vi "Remove Messages and Subaddresses.vi"(8 "error in":errorcluster, 11 "messages or subaddresses":T1[](array[typedef]) format="%.0x") -> (0 "error out":errorcluster)   [LabVIEW 2020, in "AIM MIL-STD-1553 Scripting.lvlib"]
doc: "Removes the specified <b>messages or subaddresses</b> from their parent system definition. Once the references have been removed, they are no longer valid. This VI will return an error if called to remove invalid references."
uses:
  AIM MIL-STD-1553 Scripting.lvlib
  <vilib>/NI VeriStand/Custom Device API/Custom Device Item Ref.ctl
  <vilib>/NI VeriStand/Custom Device API/Custom Device API.lvlib
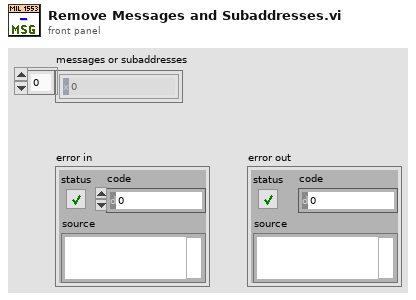
[diagram p1: front panel]
types:
  T1 = typedef "Custom Device API.lvlib/Custom Device Item Ref.ctl" = u64
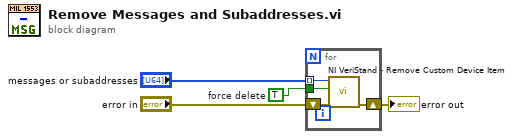
[diagram p0: block diagram]
diagram:
  w4 = TRUE  # force delete
  n1 = for {
    tunnel: w4 -> [w8]
    tunnel: "messages or subaddresses" -> [w5] mode=indexing
    shift-right: [w6] -> w2
    shift-left: "error in" -> [w7]
    n2 = call <vilib>:"NI VeriStand - Remove Custom Device Item.vi"("error in (no error)"=w7, "Force Delete (F)"=w8, "Item Ref in"=w5) -> ("error out"=w6:errorcluster)  [unwired: 7 in, 1 out]
  }
  "error out" <- w2
